vi "Response - Get, Set Header.vi"() -> (3 "Unit Test Framework Results":T1)   [LabVIEW 2017, in "Response.lvclass"]
doc: "Use this template to create a user-defined test VI. Define your test requirements and wire the results to the <b>Result (Test)</b> control. Do not modify the <b>Unit Test Framework Results</b> indicator."
uses:
  Response.lvclass
  <vilib>/utf/common/utf_test_comparison_operators.ctl
  <vilib>/utf/NI_UnitTestFramework.lvlib
  <vilib>/utf/common/utf_test_result.ctl
  <vilib>/utf/common/utf_test_result_failure.ctl
  <vilib>/utf/common/utf_test_result_troll.ctl
  <vilib>/utf/common/utf_vi_tag.ctl
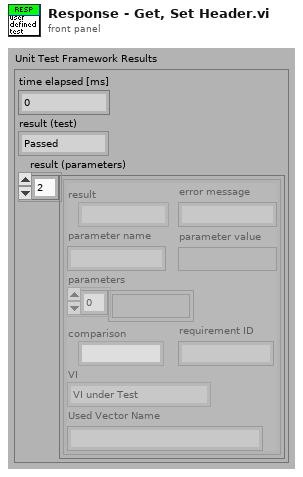
[diagram p1: front panel]
types:
  T1 = typedef "NI_UnitTestFramework.lvlib/utf_test_result_troll.ctl" = cluster{"time elapsed [ms]":u32, "result (test)":T2, "result (parameters)":T3[]}
  T2 = typedef "NI_UnitTestFramework.lvlib/utf_test_result.ctl" = enum16{"Passed", "Failed", "Error", "Skipped", "Not Processed"}
  T3 = typedef "NI_UnitTestFramework.lvlib/utf_test_result_failure.ctl" = cluster{"result":T2, "error message":string, "parameter name":string, "parameter value":variant, "parameters":variant[], "comparison":T4, "requirement ID":string, "VI":T5, "Used Vector Name":string}
  T4 = typedef "NI_UnitTestFramework.lvlib/utf_test_comparison_operators.ctl" = enum16{"=", "!=", ">", ">=", "<", "<=", "range", "symmetric tolerance", "asymmetric tolerance", "string contains", "string not contain", "array size", "string length", "array range", "by element", "array range (limit array)", "user-defined", "array contains", "array not contain", "vector length", "= (elm)", "!= (elm)", "= (case insensitive)", "!= (case insensitive)"}
  T5 = typedef "NI_UnitTestFramework.lvlib/utf_vi_tag.ctl" = enum16{"Setup VI", "VI under Test", "Teardown VI"}
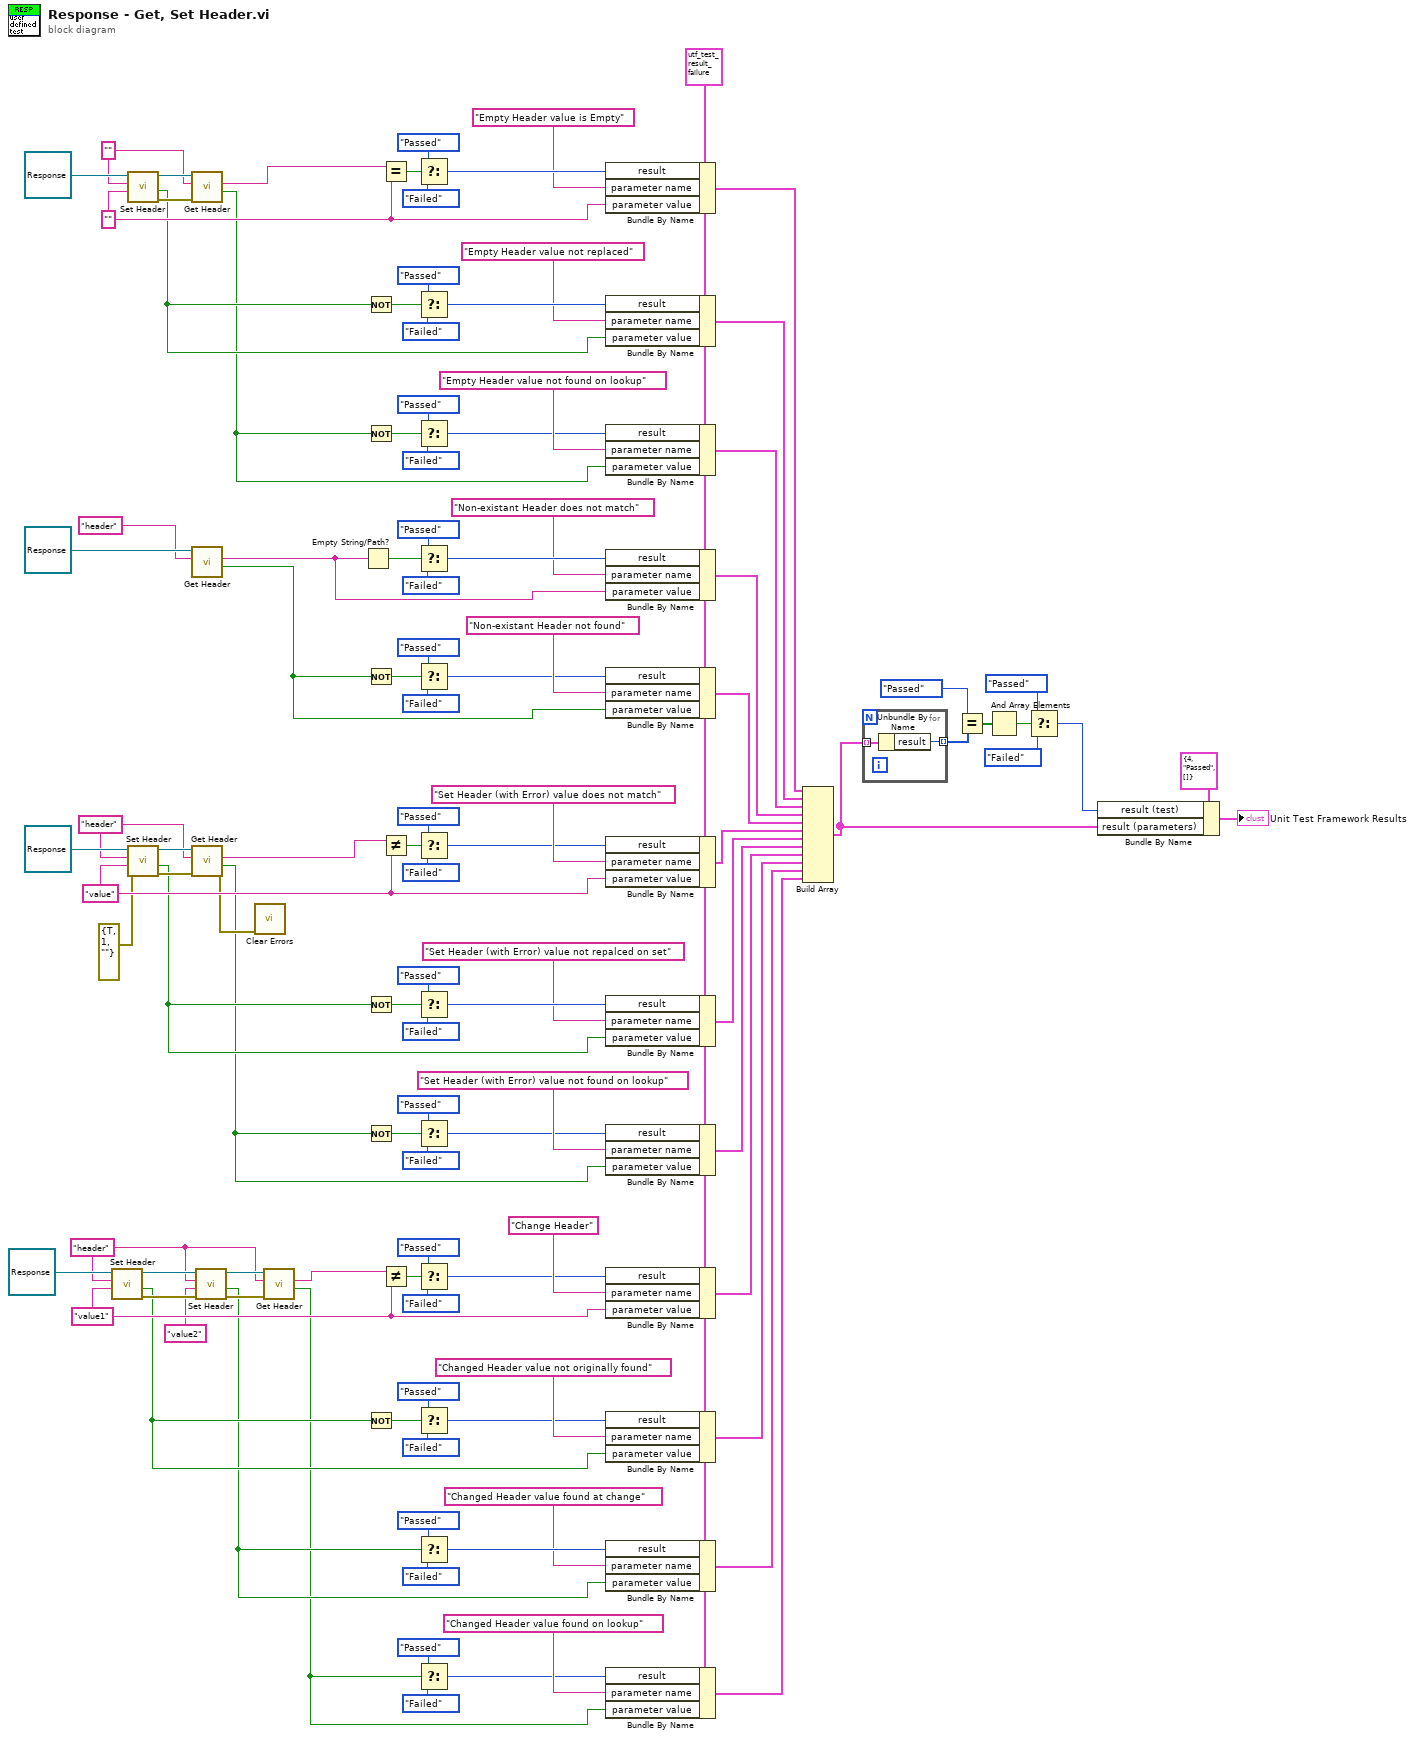
[diagram p0: block diagram]
diagram:
  w74 = "value1" ("parameter name")
  w62 = "header" ("parameter name")
  w78 = "value" ("parameter name")
  w80 = "header" ("parameter name")
  w85 = "" ("parameter name")
  w87 = "" ("parameter name")
  w2 = T3 {"result"=enum."Not Processed", "error message"="", "parameter name"="", "parameter value"=variant, "parameters"=[], "comparison"=enum."=", "requirement ID"="", "VI"=enum."VI under Test", "Used Vector Name"=""} ("Unit Test Framework - result (parameters)")
  n1 = call "Set Header.vi"("Value"=w74, "Header"=w62, "Response in"=refnum<class "Response.lvclass"> refnum) -> ("error out"=w71:errorcluster, "Replaced?"=w32:bool, "Response out"=w64:refnum<class "Response.lvclass">)  [unwired: 6 in]
  n2 = call "Set Header.vi"("Value"=w85, "Header"=w87, "Response in"=refnum<class "Response.lvclass"> refnum) -> ("error out"=w89:errorcluster, "Replaced?"=w50:bool, "Response out"=w88:refnum<class "Response.lvclass">)  [unwired: 6 in]
  n3 = call "Set Header.vi"("error in (no error)"=errorcluster {"status"=TRUE, "code"=1, "source"=""}, "Value"=w78, "Header"=w80, "Response in"=refnum<class "Response.lvclass"> refnum) -> ("error out"=w82:errorcluster, "Replaced?"=w17:bool, "Response out"=w81:refnum<class "Response.lvclass">)  [unwired: 5 in]
  n4 = call "Get Header.vi"("error in (no error)"=w89, "Header"=w87, "Response in"=w88) -> ("Found?"=w49:bool, "Value"=w86:string)  [unwired: 5 in, 2 out]
  n5 = call "Get Header.vi"("Header"="header" ("parameter name"), "Response in"=refnum<class "Response.lvclass"> refnum) -> ("Found?"=w4:bool, "Value"=w3:string)  [unwired: 6 in, 2 out]
  n6 = call "Get Header.vi"("error in (no error)"=w82, "Header"=w80, "Response in"=w81) -> ("error out"=w77:errorcluster, "Found?"=w16:bool, "Value"=w79:string)  [unwired: 5 in, 1 out]
  n7 = call "Set Header.vi"("error in (no error)"=w71, "Value"="value2" ("parameter name"), "Header"=w62, "Response in"=w64) -> ("error out"=w65:errorcluster, "Replaced?"=w31:bool, "Response out"=w63:refnum<class "Response.lvclass">)  [unwired: 5 in]
  n8 = call <vilib>:"Clear Errors.vi"("error in (no error)"=w77) -> ()  [unwired: 5 in, 2 out]
  n9 = call "Get Header.vi"("error in (no error)"=w65, "Header"=w62, "Response in"=w63) -> ("Found?"=w30:bool, "Value"=w73:string)  [unwired: 5 in, 2 out]
  n10 = Empty String/Path?(string/path=w3) -> (empty?=w5:bool)
  n11 = Not(x=w50) -> (.not. x?=w51:bool)
  n12 = Not(x=w49) -> (.not. x?=w12:bool)
  n13 = Not(x=w4) -> (.not. x?=w10:bool)
  n14 = Not(x=w17) -> (.not. x?=w18:bool)
  n15 = Not(x=w16) -> (.not. x?=w15:bool)
  n16 = Not(x=w32) -> (.not. x?=w45:bool)
  n17 = Equal?(x=w86, y=w85) -> (x = y?=w113:bool)
  n18 = Not Equal?(x=w79, y=w78) -> (x != y?=w94:bool)
  n19 = Not Equal?(x=w73, y=w74) -> (x != y?=w69:bool)
  n20 = Select(t=utf_test_result."Passed" ("result"), s=w113, f=utf_test_result."Failed" ("result")) -> (s? t:f=w112:T2)
  n21 = Select(t=utf_test_result."Passed" ("result"), s=w51, f=utf_test_result."Failed" ("result")) -> (s? t:f=w57:T2)
  n22 = Select(t=utf_test_result."Passed" ("result"), s=w12, f=utf_test_result."Failed" ("result")) -> (s? t:f=w54:T2)
  n23 = Select(t=utf_test_result."Passed" ("result"), s=w5, f=utf_test_result."Failed" ("result")) -> (s? t:f=w99:T2)
  n24 = Select(t=utf_test_result."Passed" ("result"), s=w10, f=utf_test_result."Failed" ("result")) -> (s? t:f=w8:T2)
  n25 = Select(t=utf_test_result."Passed" ("result"), s=w94, f=utf_test_result."Failed" ("result")) -> (s? t:f=w93:T2)
  n26 = Select(t=utf_test_result."Passed" ("result"), s=w18, f=utf_test_result."Failed" ("result")) -> (s? t:f=w24:T2)
  n27 = Select(t=utf_test_result."Passed" ("result"), s=w15, f=utf_test_result."Failed" ("result")) -> (s? t:f=w21:T2)
  n28 = Select(t=utf_test_result."Passed" ("result"), s=w69, f=utf_test_result."Failed" ("result")) -> (s? t:f=w68:T2)
  n29 = Select(t=utf_test_result."Passed" ("result"), s=w45, f=utf_test_result."Failed" ("result")) -> (s? t:f=w39:T2)
  n30 = Select(t=utf_test_result."Passed" ("result"), s=w31, f=utf_test_result."Failed" ("result")) -> (s? t:f=w42:T2)
  n31 = Select(t=utf_test_result."Passed" ("result"), s=w30, f=utf_test_result."Failed" ("result")) -> (s? t:f=w35:T2)
  n32 = Bundle By Name(cluster=w2, "result"=w112, "parameter name"="Empty Header value is Empty", "parameter value"=w85) -> (w46:T3)
  n33 = Bundle By Name(cluster=w2, "result"=w57, "parameter name"="Empty Header value not replaced", "parameter value"=w50) -> (w47:T3)
  n34 = Bundle By Name(cluster=w2, "result"=w54, "parameter name"="Empty Header value not found on lookup", "parameter value"=w49) -> (w48:T3)
  n35 = Bundle By Name(cluster=w2, "result"=w99, "parameter name"="Non-existant Header does not match", "parameter value"=w3) -> (w98:T3)
  n36 = Bundle By Name(cluster=w2, "result"=w8, "parameter name"="Non-existant Header not found", "parameter value"=w4) -> (w1:T3)
  n37 = Bundle By Name(cluster=w2, "result"=w93, "parameter name"="Set Header (with Error) value does not match", "parameter value"=w78) -> (w75:T3)
  n38 = Bundle By Name(cluster=w2, "result"=w24, "parameter name"="Set Header (with Error) value not repalced on set", "parameter value"=w17) -> (w14:T3)
  n39 = Bundle By Name(cluster=w2, "result"=w21, "parameter name"="Set Header (with Error) value not found on lookup", "parameter value"=w16) -> (w13:T3)
  n40 = Bundle By Name(cluster=w2, "result"=w68, "parameter name"="Change Header", "parameter value"=w74) -> (w60:T3)
  n41 = Bundle By Name(cluster=w2, "result"=w39, "parameter name"="Changed Header value not originally found", "parameter value"=w32) -> (w29:T3)
  n42 = Bundle By Name(cluster=w2, "result"=w42, "parameter name"="Changed Header value found at change", "parameter value"=w31) -> (w28:T3)
  n43 = Bundle By Name(cluster=w2, "result"=w35, "parameter name"="Changed Header value found on lookup", "parameter value"=w30) -> (w27:T3)
  n44 = Build Array(w46, w47, w48, w98, w1, w75, w14, w13, w60, w29, w28, w27) -> (w109:T3[])
  n45 = for {
    tunnel: w109 -> [w117] mode=indexing
    tunnel: [w116] -> w108 mode=indexing
    n46 = Unbundle By Name(w117) -> ("result"=w116:T2)
  }
  n47 = Equal?(x=utf_test_result."Passed" ("result"), y=w108) -> (x = y?=w106:bool[])
  n48 = And Array Elements(Boolean array=w106) -> (logical AND=w105:bool)
  n49 = Select(t=utf_test_result."Passed" ("result"), s=w105, f=utf_test_result."Failed" ("result")) -> (s? t:f=w102:T2)
  n50 = Bundle By Name(cluster=T1 {"time elapsed [ms]"=4, "result (test)"=enum."Passed", "result (parameters)"=[]} ("Unit Test Framework - Result"), "result (test)"=w102, "result (parameters)"=w109) -> (→"Unit Test Framework Results":T1)
